vi "Sense.vi"(0 "Enum":enum16{"Running", "Impact", "Spinning", "Clear"}(ring)) -> ()   [LabVIEW 2010]
uses:
  Main Global.vi
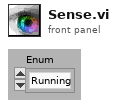
[diagram p1: front panel]
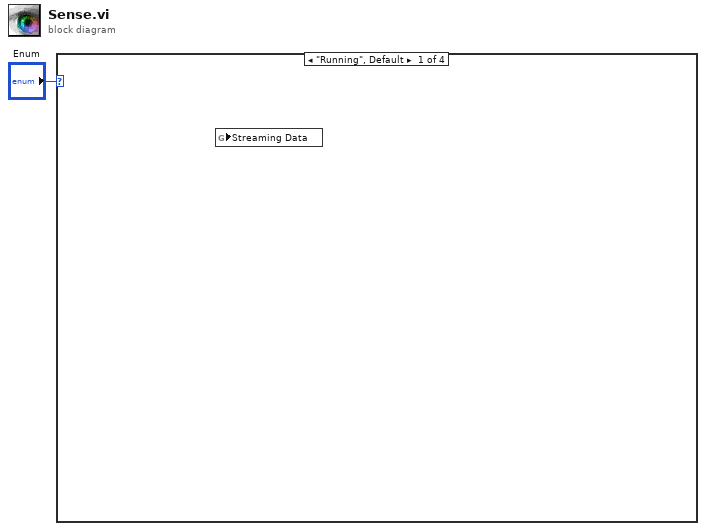
[diagram p0: block diagram]
diagram:
  n1 = case shown="\"Running\", Default" "Enum" {
    frame "Running", Default {
      n2 = global read "Main Global.vi" "Streaming Data"() -> ()  [unwired: 1 in]
    }
    frame "Impact" {
    }
    frame "Spinning" {
    }
    frame "Clear" {
    }
  }
